vi "Gas Thermal Check Tolerance.vi"(0 "Target RTDout-RTDin in":dbl, 1 "Target RTDout":dbl, 3 "Target Inlet Temperature (F)":dbl, 5 "Temperature +- Tolerance (F)":dbl, 11 "error in (no error)":errorcluster, 12 "RTDOut-RTDin Delta":dbl[](array[numeric]), 13 "RTDout":dbl[](array[numeric]), 14 "RTDin":dbl[](array[numeric])) -> (4 "RTDOut-RTDin (Max-Min) - Bool":bool, 6 "RTDout (Max-Min) Bool":bool, 8 "RTDout >= Target":bool, 10 "RTDin (Max-Min) Bool":bool, 15 "error out":errorcluster)   [LabVIEW 2020]
panel:
  out "RTDin (Min)":dbl
  out "RTDin (Max)":dbl
  out "RTDout (Min)":dbl
  out "RTDout (Max)":dbl
  out "RTDOut-RTDin (Min)":dbl
  out "RTDOut-RTDin (Max)":dbl
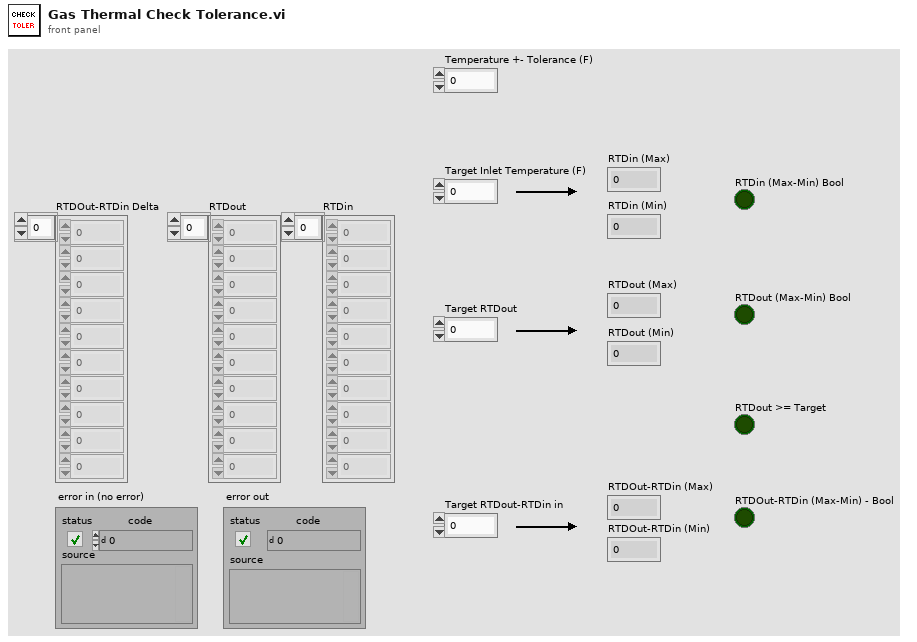
[diagram p1: front panel]
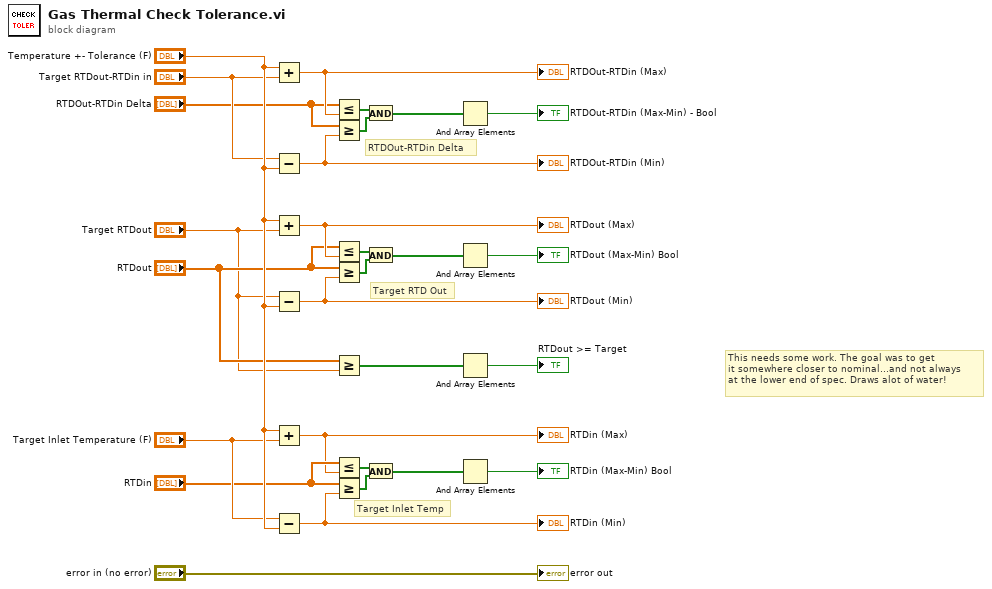
[diagram p0: block diagram]
diagram:
  # "This needs some work. The goal was to get\nit somewhere closer to nominal...and not always\nat the lower end of spec. Draws alot of water!"
  # "Target RTD Out"
  # "Target Inlet Temp"
  # "RTDOut-RTDin Delta"
  n1 = Add(x="Temperature +- Tolerance (F)", y="Target RTDout-RTDin in") -> (x+y=w22:dbl)
  "RTDOut-RTDin (Max)" <- w22
  n2 = Subtract(x="Target RTDout-RTDin in", y="Temperature +- Tolerance (F)") -> (x-y=w20:dbl)
  "RTDOut-RTDin (Min)" <- w20
  n3 = Add(x="Temperature +- Tolerance (F)", y="Target RTDout") -> (x+y=w14:dbl)
  "RTDout (Max)" <- w14
  n4 = Subtract(x="Target RTDout", y="Temperature +- Tolerance (F)") -> (x-y=w13:dbl)
  "RTDout (Min)" <- w13
  n5 = Add(x="Temperature +- Tolerance (F)", y="Target Inlet Temperature (F)") -> (x+y=w8:dbl)
  "RTDin (Max)" <- w8
  n6 = Subtract(x="Target Inlet Temperature (F)", y="Temperature +- Tolerance (F)") -> (x-y=w7:dbl)
  "RTDin (Min)" <- w7
  n7 = Less Or Equal?(x="RTDOut-RTDin Delta", y=w22) -> (x <= y?=w19:bool[])
  n8 = Greater Or Equal?(x="RTDOut-RTDin Delta", y=w20) -> (x >= y?=w18:bool[])
  n9 = Less Or Equal?(x="RTDout", y=w14) -> (x <= y?=w15:bool[])
  n10 = Greater Or Equal?(x="RTDout", y=w13) -> (x >= y?=w16:bool[])
  n11 = Greater Or Equal?(x="RTDout", y="Target RTDout") -> (x >= y?=w3:bool[])
  n12 = Less Or Equal?(x="RTDin", y=w8) -> (x <= y?=w11:bool[])
  n13 = Greater Or Equal?(x="RTDin", y=w7) -> (x >= y?=w10:bool[])
  n14 = And(x=w19, y=w18) -> (x .and. y?=w17:bool[])
  n15 = And(x=w15, y=w16) -> (x .and. y?=w12:bool[])
  n16 = And(x=w11, y=w10) -> (x .and. y?=w6:bool[])
  n17 = And Array Elements(Boolean array=w17) -> (logical AND=→"RTDOut-RTDin (Max-Min) - Bool":bool)
  n18 = And Array Elements(Boolean array=w12) -> (logical AND=→"RTDout (Max-Min) Bool":bool)
  n19 = And Array Elements(Boolean array=w3) -> (logical AND=→"RTDout >= Target":bool)
  n20 = And Array Elements(Boolean array=w6) -> (logical AND=→"RTDin (Max-Min) Bool":bool)
  "error out" <- "error in (no error)"
